vi "Select multiplexer LR700.vi"(8 "error in":errorcluster, 10 "Sensor":i32, 11 "VISA Resource Name":refnum<visa-resource-name>) -> (0 "error out":errorcluster, 3 "VISA Resource Name Out":refnum<visa-resource-name>)   [LabVIEW 2019]
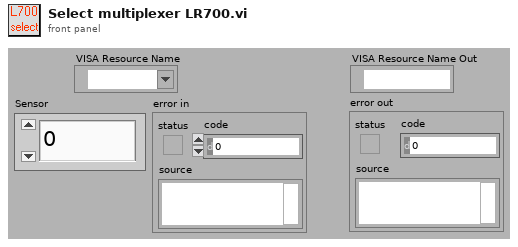
[diagram p1: front panel]
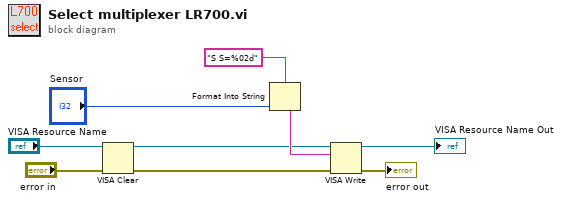
[diagram p0: block diagram]
diagram:
  n1 = VISA Clear(VISA resource name="VISA Resource Name", error in (no error)="error in") -> (VISA resource name out=w3:refnum<visa-resource-name>, error out=w5:errorcluster)
  n2 = Format Into String(format string="S S=%02d", "Sensor") -> (resulting string=w8:string)  [unwired: 2 in, 1 out]
  n3 = VISA Write(VISA resource name=w3, write buffer=w8, error in (no error)=w5) -> (VISA resource name out=→"VISA Resource Name Out":refnum<visa-resource-name>, error out=→"error out":errorcluster)  [unwired: 1 out]
